vi "RT_control_ref_test_v1.vi"() -> ()   [LabVIEW 2011]
panel:
  in  "t":dbl
  in  "W_b(i) [rad/s]":dbl[](array[numeric])
  in  "Euler Angles [rad]":dbl[](array[numeric])
  out "TVA_cmd [rad]":dbl[](array[numeric])
  in  "TVA_y [º]":dbl format="%#_13g"
  in  "TVA_p [º]":dbl format="%#_13g"
  out "TVA_b":dbl[](array[numeric])
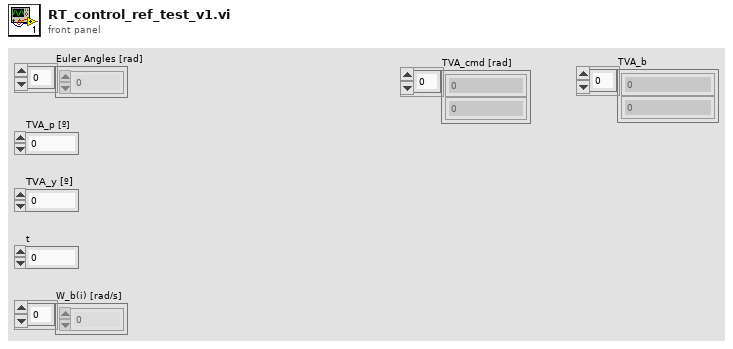
[diagram p1: front panel]
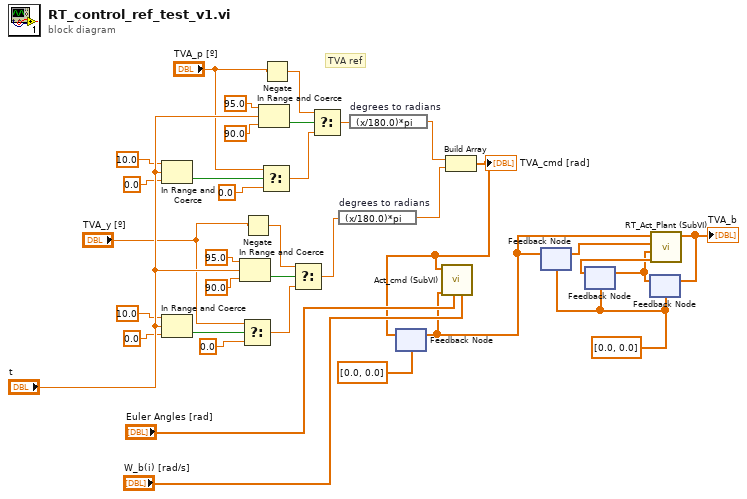
[diagram p0: block diagram]
diagram:
  w2 = dbl[] [0.0, 0.0] ("TVA_b")
  # "TVA ref"
  n1 = In Range and Coerce(upper limit=10.0, x="t", lower limit=0.0) -> (In Range?=w13:bool)  [unwired: 1 out]
  n2 = In Range and Coerce(upper limit=10.0, x="t", lower limit=0.0) -> (In Range?=w25:bool)  [unwired: 1 out]
  n3 = In Range and Coerce(upper limit=95.0, x="t", lower limit=90.0) -> (In Range?=w26:bool)  [unwired: 1 out]
  n4 = Select(t="TVA_y [º]", s=w25, f=0.0 ("t")) -> (s? t:f=w27:dbl)
  n5 = Negate(x="TVA_y [º]") -> (-x=w28:dbl)
  n6 = In Range and Coerce(upper limit=95.0, x="t", lower limit=90.0) -> (In Range?=w12:bool)  [unwired: 1 out]
  n7 = Select(t="TVA_p [º]", s=w13, f=0.0 ("t")) -> (s? t:f=w10:dbl)
  n8 = Negate(x="TVA_p [º]") -> (-x=w7:dbl)
  n9 = Select(t=w28, s=w26, f=w27) -> (s? t:f=w30:dbl)
  n10 = Select(t=w7, s=w12, f=w10) -> (s? t:f=w11:dbl)
  n11 = expression code="(x/180.0)*pi" "degrees to radians"(w30) -> (w8:dbl)
  n12 = expression code="(x/180.0)*pi" "degrees to radians"(w11) -> (w9:dbl)
  n13 = feedback #1(dbl[] [0.0, 0.0] ("TVA_cmd")) -> (w33:dbl[])
  n14 = Build Array(w9, w8) -> (w32:dbl[])
  "TVA_cmd [rad]" <- w32
  n15 = feedback-in #1(w32) -> ()
  n16 = call "Act_cmd (SubVI).vi"("W_b [rad/s]"="W_b(i) [rad/s]", "Angles [rad]"="Euler Angles [rad]", "TVA_old [rad]"=w33, "TVA_cmd [rad]"=w32) -> ()  [unwired: 6 in, 2 out]
  n17 = feedback #2(w2) -> (w3:dbl[])
  n18 = feedback-in #2(w33) -> ()
  n19 = feedback #3(w2) -> (w6:dbl[])
  n20 = feedback #4(w2) -> (w5:dbl[])
  n21 = feedback-in #3(w5) -> ()
  n22 = call "RT_Act_Plant (SubVI).vi"("Act_b(i-2)"=w6, "Act_b(i-1)"=w5, "Act_cmd (i-2) [rad]"=w3, "Act_cmd (i-1) [rad]"=w33) -> ("Act_b"=w4:dbl[])  [unwired: 7 in]
  "TVA_b" <- w4
  n23 = feedback-in #4(w4) -> ()
